vi "Script Con And Wire.vi"(4 "VI Name":string, 6 "Indicator":bool, 8 "error in":errorcluster, 9 "VI":refnum<vi>, 10 "Terminal Attributes":T1) -> (0 "error out":errorcluster)   [LabVIEW 2020, in "_Rescript.lvlib"]
uses:
  _Rescript.lvlib
  Attributes.ctl
  Terminal Attributes.ctl
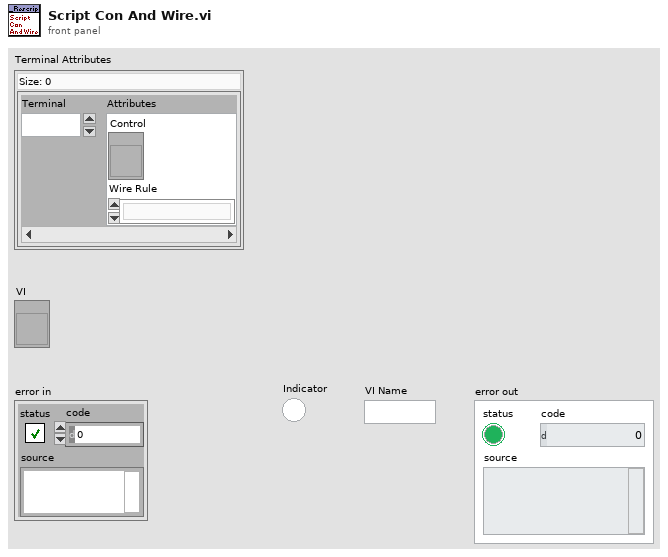
[diagram p1: front panel]
types:
  T1 = typedef "_Rescript.lvlib/Terminal Attributes.ctl" = map{i32, T2}
  T2 = typedef "_Rescript.lvlib/Attributes.ctl" = cluster{"Control":refnum<vi>, "Wire Rule":enum16{"Invalid Wire Rule", "Required", "Recommended", "Optional", "Dynamic Dispatch"}}
  T3 = enum16{"Invalid Wire Rule", "Required", "Recommended", "Optional", "Dynamic Dispatch"}
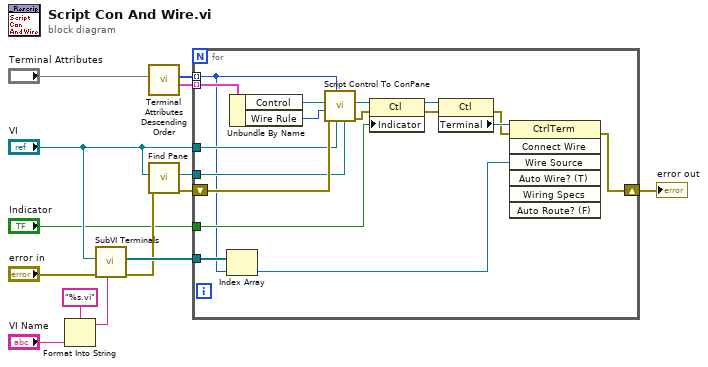
[diagram p0: block diagram]
diagram:
  n1 = Format Into String(format string="%s.vi", "VI Name") -> (resulting string=w1:string)  [unwired: 2 in, 1 out]
  n2 = call "SubVI Terminals.vi"("Label"=w1, "error in"="error in", "VI"="VI") -> ("error out"=w9:errorcluster, "Terminals[]"=w10:refnum<vi>[])  [unwired: 7 in]
  n3 = call "Terminal Attributes Descending Order.vi"("Terminal Attributes"="Terminal Attributes") -> ("Attributes Descending Order"=w12:T2[], "Terminal Descending Order"=w11:i32[])  [unwired: 9 in]
  n4 = call "Find Pane.vi"("error in"=w9, "VI"="VI") -> ("error out"=w14:errorcluster, "Pane Ref"=w13:refnum<vi>)  [unwired: 8 in]
  n5 = for {
    tunnel: w11 -> [w15] mode=indexing
    tunnel: w13 -> [w27]
    tunnel: "VI" -> [w21]
    shift-right: [w29] -> w5
    shift-left: w14 -> [w28]
    tunnel: w12 -> [w19] mode=indexing
    tunnel: "Indicator" -> [w18]
    tunnel: w10 -> [w17]
    n6 = Index Array(array=w17, index=w15) -> (element=w16:refnum<vi>)
    n7 = Unbundle By Name(w19) -> ("Control"=w26:refnum<vi>, "Wire Rule"=w25:T3)
    n8 = call "Script Control To ConPane.vi"("Pane"=w27, "VI"=w21, "Terminal"=w15, "error in"=w28, "Wire Rule"=w25, "Control To Duplicate"=w26) -> ("error out"=w23:errorcluster, "Duplicated Control"=w24:refnum<vi>)  [unwired: 4 in]
    n9 = property class="Ctl"(reference=w24, error in=w23, "Indicator"=w18) -> (reference out=w22:refnum<vi>, error out=w20:errorcluster)
    n10 = property class="Ctl"(reference=w22, error in=w20) -> (error out=w30:errorcluster, "Terminal"=w31:refnum<vi>)  [unwired: 1 out]
    n11 = invoke class="CtrlTerm" method="Connect Wire"(reference=w31, error in=w30, "Wire Source"=w16) -> (error out=w29:errorcluster)  [unwired: 4 in, 6 out]
  }
  "error out" <- w5
